vi "Read Serial Port Attributes.vi"(8 "error in (no error)":errorcluster, 11 "SerialDriver in":refnum<class "SerialDriver.lvclass">) -> (0 "error out":errorcluster, 2 "Serial Port Attributes":T1={"Baud Rate"=9600, "Data Bits"=8, "Stop Bits"=10, "Data Flow"=0, "Timeout"=0, "parity (0:none)"=enum."None", "Establish Wait"=10000} {"Stop Bits" items=["1.0"=10, "1.5"=15, "2.0"=20]}, 3 "SerialDriver out":refnum<class "SerialDriver.lvclass">)   [LabVIEW 2023, in "HAF.lvlib" / "SerialDriver.lvclass"]
doc: "Returns the attributes to use to configure the Serial Port used by this Driver."
uses:
  SerialDriver.lvclass
  Serial Port Attributes.ctl
  HAF.lvlib
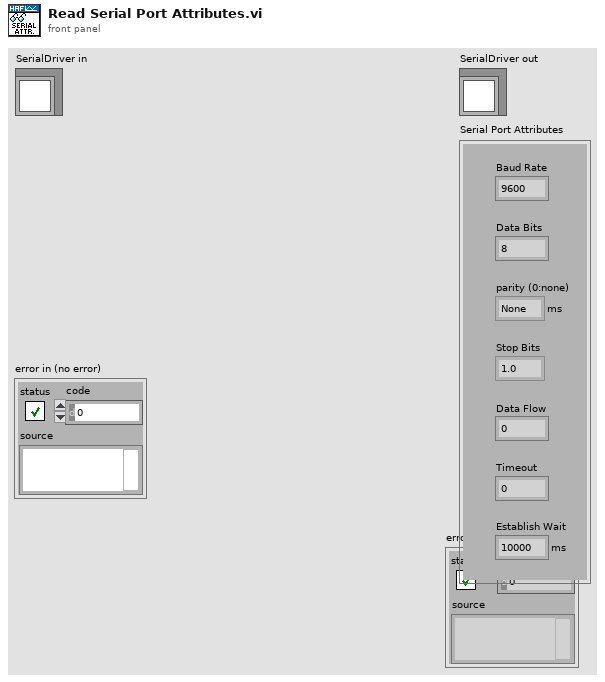
[diagram p1: front panel]
types:
  T1 = typedef "HAF.lvlib/Serial Port Attributes.ctl" = cluster{"Baud Rate":u32, "Data Bits":u16, "Stop Bits":u16, "Data Flow":u16, "Timeout":u32, "parity (0:none)":enum16{"None", "Odd", "Even", "Mark", "Space"}, "Establish Wait":u32}
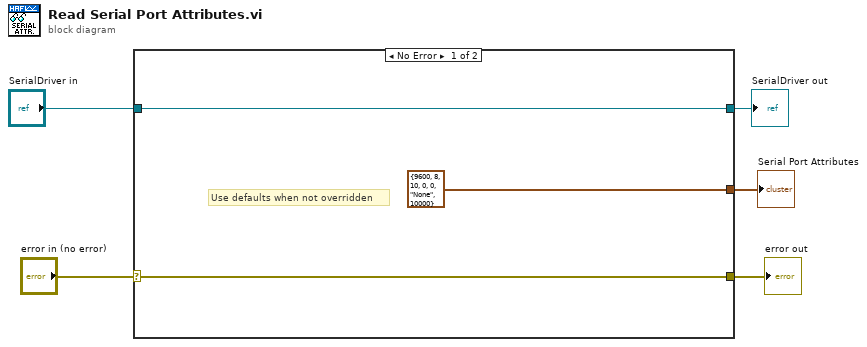
[diagram p0: block diagram]
diagram:
  n1 = case shown="No Error" "error in (no error)" {
    selector: "error in (no error)" -> [w7 w10]
    tunnel: [w7 w10] -> w4
    tunnel: [w8 w9] -> w2
    tunnel: "SerialDriver in" -> [w8 w9]
    tunnel: [T1 {"Baud Rate"=9600, "Data Bits"=8, "Stop Bits"=10, "Data Flow"=0, "Timeout"=0, "parity (0:none)"=enum."None", "Establish Wait"=10000} ("Serial Port Attributes") _] -> w1
    frame No Error {
      # "Use defaults when not overridden"
    }
    frame Error {
    }
  }
  "error out" <- w4
  "SerialDriver out" <- w2
  "Serial Port Attributes" <- w1
